vi "Periodic Tasks.vi"(8 "error in":errorcluster) -> ()   [LabVIEW 2017]
doc: "This VI runs in parallel to other tasks. It can contain as many user-defined periodic loops as you need. These can carry out PID or other sorts of timed response."
uses:
  <vilib>/Rock Robotics/WPI/DriverStation/WPI_DriverStationRobotMode2.ctl
  <vilib>/Rock Robotics/WPI/Utilities/WPI_GetSetVariantRefNum.vi
  Robot Global Data.vi
  <vilib>/Rock Robotics/WPI/RobotDrive/WPI_RobotDriveArcadeDrive_Standard(NoSaturation).vi
  <vilib>/Rock Robotics/Network Tables/NT Write Numeric Array.vi
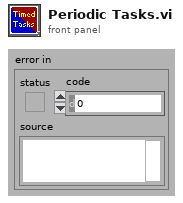
[diagram p1: front panel]
types:
  T1 = typedef "WPI_JoystickDevRef.ctl" = cluster{"Device":T2}
  T2 = typedef "WPI_JoystickDeviceEnum.ctl" = enum16{"USB 0", "USB 1", "USB 2", "USB 3", "USB 4", "USB 5"}
  T3 = typedef "WPI_RobotDriveDevRef.ctl" = cluster{"DevStatus":errorcluster, "Motors[]":T4[], "Square Inputs":bool, "Max Output":dbl}
  T4 = typedef "WPI_MotorControlDeviceRef.ctl" = cluster{"DeviceStatus":errorcluster, "Type":T5, "PWM":cluster{"PWM Channel":T6, "DeadBand":T7}, "CAN":cluster{"Device Number":u8, "SetOutput VI Ref":variant, "GetOutput VI Ref":variant, "Enable VI Ref":variant, "Disable VI Ref":variant, "Data":variant}, "Invert":bool, "DIO PWM":cluster{"PWM \"Enable\" Channel":T6, "DIOChannel":T8, "PWM Rate":dbl}}
  T5 = typedef "WPI_MotorControlType.ctl" = enum16{"PWM", "CAN", "DIO PWM"}
  T6 = typedef "FPGA_DIOPWMChannel.ctl" = enum8{"PWM 0", "PWM 1", "PWM 2", "PWM 3", "PWM 4", "PWM 5", "PWM 6", "PWM 7", "PWM 8", "PWM 9", "PWM MXP 0", "PWM MXP 1", "PWM MXP 2", "PWM MXP 3", "PWM MXP 4", "PWM MXP 5", "PWM MXP 6", "PWM MXP 7", "PWM MXP 8", "PWM MXP 9", "Invalid"}
  T7 = typedef "WPI_PWMDeadband.ctl" = cluster{"Name":string, "maxPositivePwm":i32, "minPositivePwm":i32, "centerPwm":i32, "maxNegativePwm":i32, "minNegativePwm":i32, "angularRange":u16}
  T8 = typedef "FPGA_DIOChannel.ctl" = enum8{"DIO 0", "DIO 1", "DIO 2", "DIO 3", "DIO 4", "DIO 5", "DIO 6", "DIO 7", "DIO 8", "DIO 9", "DIO MXP 0", "DIO MXP 1", "DIO MXP 2", "DIO MXP 3", "DIO MXP 4", "DIO MXP 5", "DIO MXP 6", "DIO MXP 7", "DIO MXP 8", "DIO MXP 9", "DIO MXP 10", "DIO MXP 11", "DIO MXP 12", "DIO MXP 13", "DIO MXP 14", "DIO MXP 15", "SPI Port CS1", "SPI Port CS2", "SPI Port CS3", "SPI Port MISO", "SPI Port MOSI", "Invalid"}
  T9 = typedef "WPI_EncoderDevRef.ctl" = cluster{"DevStatus":errorcluster, "EncoderIndex":T10, "CounterIndex":T11, "DistancePerCount":dbl, "Decoding Type":T12}
  T10 = typedef "FPGA_EncoderIdx.ctl" = enum8{"Enc 0", "Enc 1", "Enc 2", "Enc 3", "Enc 4", "Enc 5", "Enc 6", "Enc 7", "Invalid"}
  T11 = typedef "FPGA_CounterCtrSystemIndex.ctl" = enum8{"Ctr 0", "Ctr 1", "Ctr 2", "Ctr 3", "Ctr 4", "Ctr 5", "Ctr 6", "Ctr 7", "Invalid"}
  T12 = typedef "WPI_EncoderType.ctl" = enum16{"1x", "2x", "4x"}
  T13 = typedef "WPI_GyroDevRef.ctl" = cluster{"DevStatus":errorcluster, "Analog Channel":T14, "Gain (VoltsPerDegree/Second)":dbl, "Gyro Type":enum16{"Analog", "XRS450"}, "Handle":i32, "SPI Bus":T15, "Device Found":bool, "Sample Rate":dbl, "Calibrate On Open":bool, "Offset":dbl}
  T14 = typedef "FPGA_AIChannel.ctl" = enum8{"AI 0", "AI 1", "AI 2", "AI 3", "AI MXP 0", "AI MXP 1", "AI MXP 2", "AI MXP 3", "Invalid"}
  T15 = typedef "spi_bus.ctl" = enum16{"SPI On-Board, CS0", "SPI On-Board, CS1", "SPI On-Board, CS2", "SPI On-Board, CS3", "SPI MXP", "Invalid"}
  T16 = cluster{"JoystickDevRef":T1, "RobotDriveDevRef":T3}
  T17 = typedef "WPI_DriverStationRobotMode2.ctl" = enum16{"Autonomous Disabled", "Autonomous Enabled", "Teleop Disabled", "Teleop Enabled", "Disconnected", "Finish", "Test Disabled", "Test Enabled", "Emergency Stopped"}
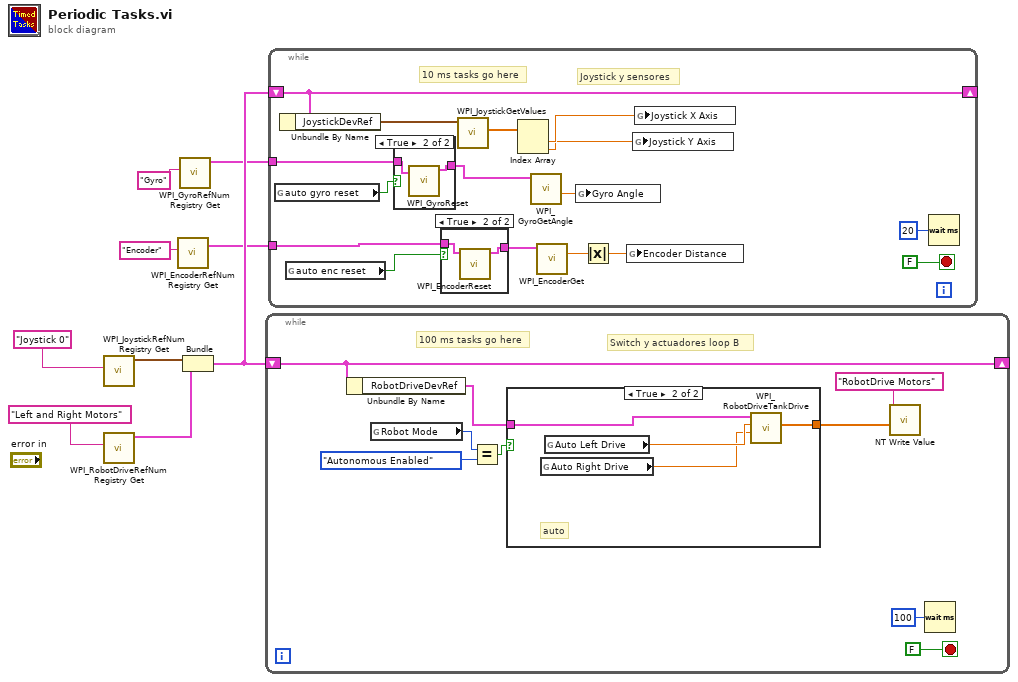
[diagram p0: block diagram]
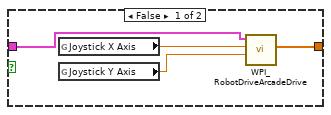
[diagram p2: hidden frame]
diagram:
  n1 = call <vilib>:"WPI_JoystickRefNum Registry Get.vi"("refnum name"="Joystick 0") -> ("JoystickDevRef"=w7:T1)  [unwired: 1 in, 9 out]
  n2 = call <vilib>:"WPI_RobotDriveRefNum Registry Get.vi"("refnum name"="Left and Right Motors") -> ("RobotDriveDevRef"=w6:T3)  [unwired: 1 in, 9 out]
  n3 = call <vilib>:"WPI_EncoderRefNum Registry Get.vi"("refnum name"="Encoder") -> ("EncoderDevRef"=w4:T9)  [unwired: 9 in, 1 out]
  n4 = call <vilib>:"WPI_GyroRefNum Registry Get.vi"("refnum name"="Gyro") -> ("GyroDevRef"=w1:T13)  [unwired: 9 in, 1 out]
  n5 = Bundle("JoystickDevRef"=w7, "RobotDriveDevRef"=w6) -> (w5:T16)  [unwired: 1 out]
  n6 = while {
    shift-right: [w16] -> _
    shift-left: w5 -> [w16]
    stop <- FALSE stop-if-true
    # "Switch y actuadores loop B"
    # "100 ms tasks go here"
    n7 = Unbundle By Name(w16) -> ("RobotDriveDevRef"=w12:T3)
    n8 = global read "Robot Global Data.vi" "Robot Mode"() -> (w14:T17)
    n9 = Equal?(x=w14, y=WPI_DriverStationRobotMode2."Autonomous Enabled") -> (x = y?=w15:bool)
    n10 = case shown="True" w15 {
      tunnel: w12 -> [w19 w26]
      tunnel: [w20 w25] -> w10
      frame False {
        n11 = global read "Robot Global Data.vi" "Joystick X Axis"() -> (w22:dbl)
        n12 = global read "Robot Global Data.vi" "Joystick Y Axis"() -> (w21:dbl)
        n13 = call-poly <vilib>:"WPI_RobotDriveArcadeDrive.vi"("Y axis value"=w21, "X axis value"=w22, "RobotDriveDevRef"=w19) -> ("Motor Values"=w20:dbl[])  [unwired: 6 in, 2 out]
      }
      frame True {
        # "auto"
        n14 = global read "Robot Global Data.vi" "Auto Right Drive"() -> (w23:dbl)
        n15 = global read "Robot Global Data.vi" "Auto Left Drive"() -> (w24:dbl)
        n16 = call <vilib>:"WPI_RobotDriveTankDrive.vi"("Right axis value"=w23, "Left axis value"=w24, "RobotDriveDevRef"=w26) -> ("Motor Values"=w25:dbl[])  [unwired: 6 in, 2 out]
      }
    }
    n17 = call-poly <vilib>:"NT Write Value.vi"("Numeric Array"=w10, "Name"="RobotDrive Motors") -> ()  [unwired: 9 in, 1 out]
    n18 = Wait (ms)(milliseconds to wait=u32 100) -> ()  [unwired: 1 out]
  }
  n19 = while {
    shift-right: [w40] -> _
    shift-left: w5 -> [w40]
    tunnel: w4 -> [w30]
    tunnel: w1 -> [w34]
    stop <- FALSE stop-if-true
    # "Joystick y sensores"
    # "10 ms tasks go here"
    n20 = global read "Robot Global Data.vi" "auto gyro reset"() -> (w32:bool)
    n21 = Unbundle By Name(w40) -> ("JoystickDevRef"=w39:T1)
    n22 = global read "Robot Global Data.vi" "auto enc reset"() -> (w29:bool)
    n23 = case shown="True" w32 {
      tunnel: w34 -> [w46 w48]
      tunnel: [w46 w47] -> w33
      frame False {
      }
      frame True {
        n24 = call <vilib>:"WPI_GyroReset.vi"("GyroDevRef"=w48) -> ("GyroDevRef"=w47:T13)  [unwired: 9 in, 1 out]
      }
    }
    n25 = case shown="True" w29 {
      tunnel: [w43 w45] -> w31
      tunnel: w30 -> [w43 w44]
      frame False {
      }
      frame True {
        n26 = call <vilib>:"WPI_EncoderReset.vi"("EncoderDevRef"=w44) -> ("EncoderDevRef"=w45:T9)  [unwired: 9 in, 1 out]
      }
    }
    n27 = call <vilib>:"WPI_JoystickGetValues.vi"("JoystickDevRef"=w39) -> ("Axes"=w38:dbl[])  [unwired: 6 in, 4 out]
    n28 = Index Array(array=w38) -> (element #1=w37:dbl, element #2=w36:dbl)  [unwired: 2 in]
    n29 = call <vilib>:"WPI_GyroGetAngle.vi"("GyroDevRef"=w33) -> ("Angular Rate"=w35:dbl)  [unwired: 7 in, 3 out]
    n30 = call <vilib>:"WPI_EncoderGet.vi"("EncoderDevRef"=w31) -> ("Distance"=w28:dbl)  [unwired: 5 in, 5 out]
    n31 = global write "Robot Global Data.vi" "Gyro Angle"(w35) -> ()
    n32 = Absolute Value(x=w28) -> (abs(x)=w27:dbl)
    n33 = global write "Robot Global Data.vi" "Encoder Distance"(w27) -> ()
    n34 = global write "Robot Global Data.vi" "Joystick Y Axis"(w36) -> ()
    n35 = global write "Robot Global Data.vi" "Joystick X Axis"(w37) -> ()
    n36 = Wait (ms)(milliseconds to wait=u32 20) -> ()  [unwired: 1 out]
  }
